vi "TC Channel Config.vi"(8 "error in (no error)":errorcluster, 11 "Node Ptr":T4 format="%.0x") -> (0 "error out":errorcluster)   [LabVIEW 2011, in "Simulated Thermocouple Custom Device.lvlib"]
uses:
  Simulated Thermocouple Custom Device.lvlib
  <vilib>/NI Veristand/Custom Device API/Custom Device Item Ref.ctl
  TC Channel Config Data.ctl
  TC Selector.ctl
  TC Unit Selector.ctl
  Calibration Config Data.ctl
  <vilib>/NI Veristand/Custom Device API/Get Item Property (Variant).vi
  <vilib>/NI Veristand/Custom Device API/Get Item Property (String).vi
  <vilib>/NI Veristand/Custom Device API/Set Item Property (String).vi
  <vilib>/NI Veristand/Custom Device API/Set Item Property (Variant).vi
  <vilib>/regexp/Match Regular Expression.xnode
  <vilib>/NI Veristand/Custom Device API/Custom Device API.lvlib
panel:
  out "Address":string
  in  "Physical Channel":u16(ring) items=["0", "1", "2", "3", "4", "5", "6", "7", "8", "9", "10", "11", "12", "13", "14", "15", "16", "17", "18", "19", "20", "21", "22", "23", "24", "25", "26", "27", "28", "29", "30", "31"]
  in  "Header 3":cluster{"Section Name":string}={"Section Name"="Physical Channel"}
  out "TC Channel Config":T1 {"Temperature Units" items=["Celcius", "Fahrenheit", "Kelvin", "Rankine", "Volts"]; "Thermocouple Type" items=["J", "K", "T", "E", "N", "B", "R", "S", "Raw Voltage"]}
  in  "Header 2":cluster{"Section Name":string}={"Section Name"="Thermocouple Settings"}
  in  "Header":cluster{"Section Name":string}={"Section Name"="Simulated Thermocouple Channel Specification"}
  in  "Description":string="This page allows you configure the type of thermocouple to simulate, and the units of the desired temperature output.  The phsyical channel below can be changed via the Physical Channel Selector."
  in  "Name":string
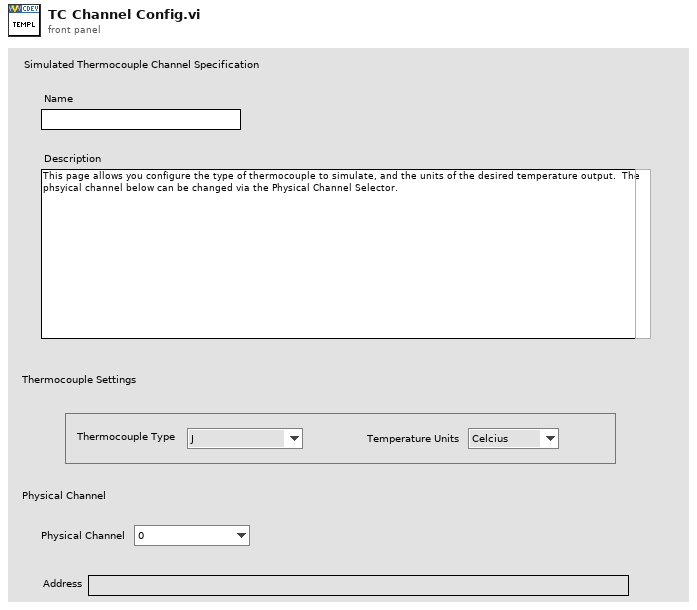
[diagram p1: front panel]
types:
  T1 = typedef "Simulated Thermocouple Custom Device.lvlib/TC Channel Config Data.ctl" = cluster{"Thermocouple Type":T2, "Temperature Units":T3}
  T2 = typedef "Simulated Thermocouple Custom Device.lvlib/TC Selector.ctl" = u16
  T3 = typedef "Simulated Thermocouple Custom Device.lvlib/TC Unit Selector.ctl" = u16
  T4 = typedef "Custom Device API.lvlib/Custom Device Item Ref.ctl" = u64
  T5 = typedef "Custom Device API.lvlib/Custom Device Item Info.ctl" = cluster{"Name":string, "Is Channel":bool, "GUID":string}
  T6 = typedef "Simulated Thermocouple Custom Device.lvlib/Calibration Config Data.ctl" = cluster{"Local SimTC Chan":string, "Samples To Collect":dbl, "Cal Channel TC Type":T2, "Cal Step Settling Time":dbl}
  T7 = typedef "Custom Device API.lvlib/Custom Device Commands.ctl" = enum16{"Default", "Item renamed", "Shutdown", "Dynamic button pressed"}
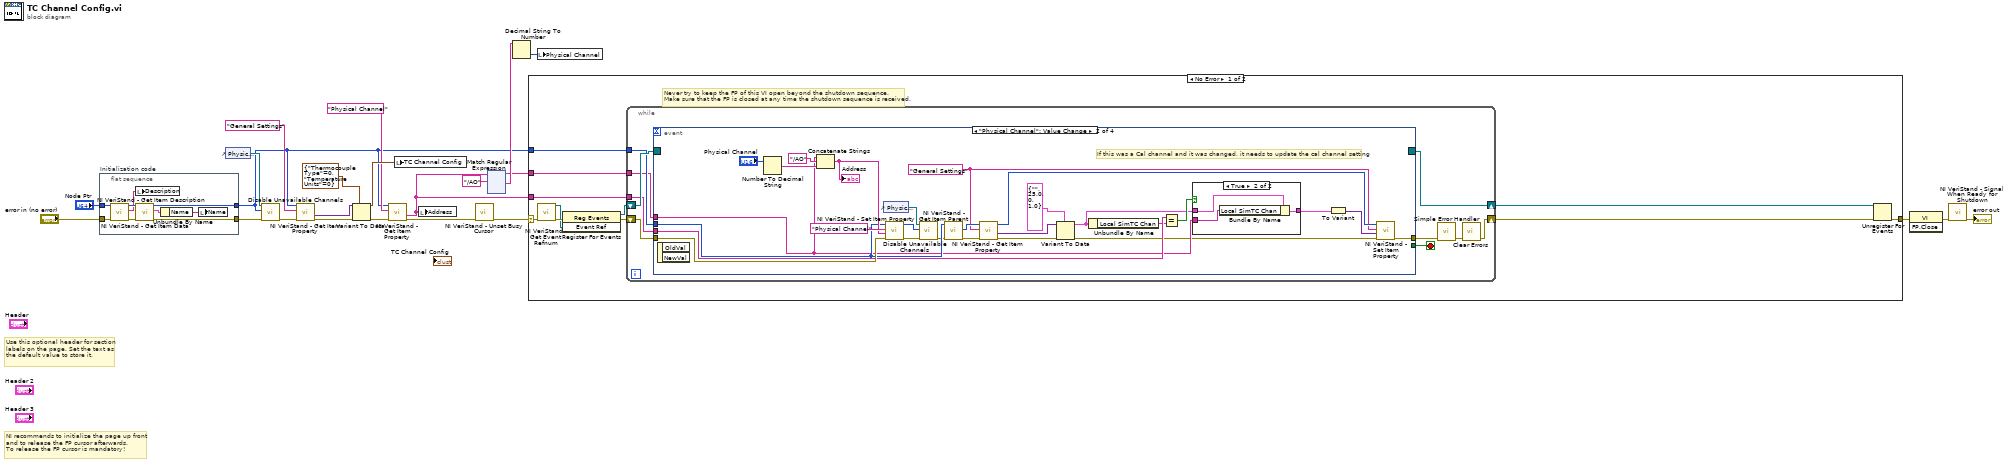
[diagram p0: block diagram]
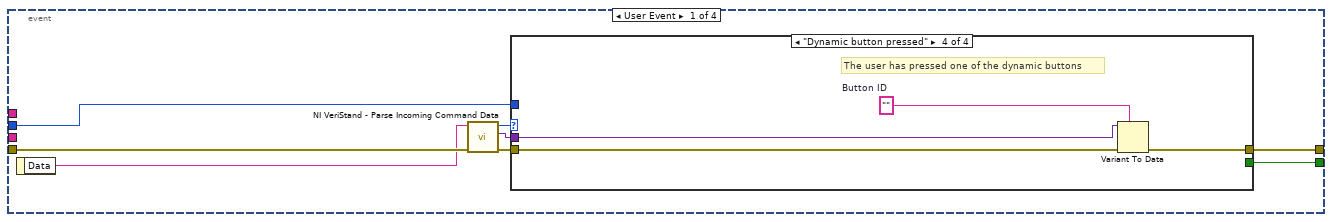
[diagram p2: hidden frame]
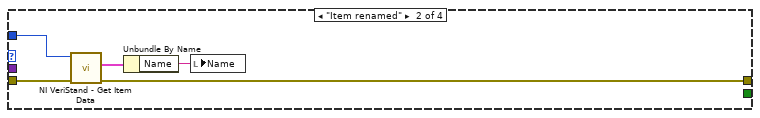
[diagram p4: hidden frame]
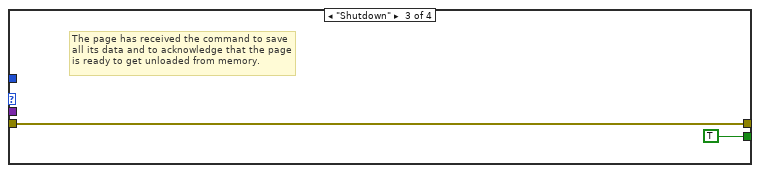
[diagram p5: hidden frame]
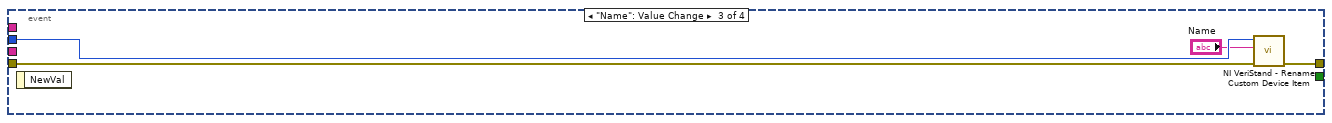
[diagram p7: hidden frame]
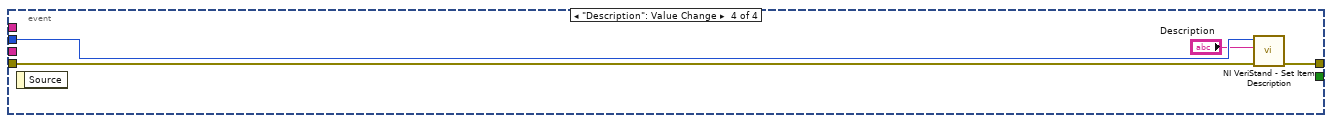
[diagram p8: hidden frame]
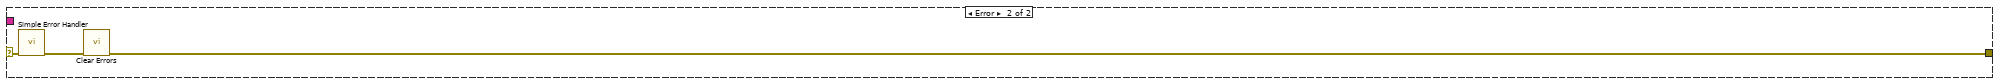
[diagram p9: hidden frame]
diagram:
  # "Use this optional header for section labels on the page. Set the text as the default value to store it."
  # "NI recommends to initialize the page up front\nand to release the FP cursor afterwards.\nTo release the FP cursor is mandatory!"
  n1 = flat-sequence "Initialization code" {
    tunnel: "error in (no error)" -> [w30]
    tunnel: "Node Ptr" -> [w29]
    tunnel: [w24] -> w17
    tunnel: [w32] -> w3
    frame #0 {
      n2 = call <vilib>:"NI VeriStand - Get Item Description.vi"("error in (no error)"=w30, "Item Ref in"=w29) -> ("error out"=w27:errorcluster, "Description"=w28:string, "Item Ref out"=w31:T4)  [unwired: 7 out]
      n3 = local write "Description"(w28) -> ()
      n4 = call <vilib>:"NI VeriStand - Get Item Data.vi"("error in (no error)"=w27, "Item Ref in"=w31) -> ("error out"=w24:errorcluster, "Item Info"=w26:T5, "Item Ref out"=w32:T4)  [unwired: 7 out]
      n5 = Unbundle By Name(w26) -> ("Name"=w25:string)
      n6 = local write "Name"(w25) -> ()
    }
  }
  n7 = control-ref of="Physical Channel"() -> (w16:refnum<vi>)
  n8 = call "Disable Unavailable Channels.vi"("error in (no error)"=w17, "Item Ref out"=w3, "Ring in"=w16) -> ("error out"=w15:errorcluster)  [unwired: 8 in]
  n9 = call-poly <vilib>:"NI VeriStand - Get Item Property.vi"("error in (no error)"=w15, "Property Name"="General Settings", "Item Ref in"=w3) -> ("error out"=w4:errorcluster, "Value"=w5:variant)  [unwired: 5 in, 2 out]
  n10 = Variant To Data(error in=w4, type=T1 {"Thermocouple Type"=0, "Temperature Units"=0} ("TC Channel Config"), Variant=w5) -> (data=w13:T1, error out=w12:errorcluster)
  n11 = call-poly <vilib>:"NI VeriStand - Get Item Property.vi"("error in (no error)"=w12, "Property Name"="Physical Channel", "Item Ref in"=w3) -> ("error out"=w8:errorcluster, "Value"=w1:string)  [unwired: 5 in, 2 out]
  n12 = local write "TC Channel Config"(w13) -> ()
  n13 = local write "Address"(w1) -> ()
  n14 = call <vilib>:"NI VeriStand - Unset Busy Cursor.vi"("error in (no error)"=w8) -> ("error out"=w19:errorcluster)  [unwired: 10 out]
  n15 = xnode "Match Regular Expression"("input string"=w1, "regular expression"="/AO") -> ("before match"=w7:string, "after match"=w10:string)  [unwired: 4 in, 3 out]
  n16 = Decimal String To Number(string=w10) -> (number=w9:i32)  [unwired: 2 in, 1 out]
  n17 = case shown="No Error" w19 {
    selector: w19 -> [w35 w115]
    tunnel: [w40 w113] -> w23
    tunnel: w3 -> [w36 _]
    tunnel: w7 -> [w34 _]
    tunnel: w1 -> [w33 _]
    frame No Error {
      # "Never try to keep the FP of this VI open beyond the shutdown sequence.\nMake sure that the FP is closed at any time the shutdown sequence is received."
      n18 = call <vilib>:"NI VeriStand - Get Event Refnum.vi"("error in (no error)"=w35) -> ("error out"=w43:errorcluster, "Event Ref"=w39:refnum<user-event>)  [unwired: 9 out]
      n19 = register-events(error in=w43, w39) -> (reference out=w37:refnum<event-registration>, error out=w38:errorcluster)  [unwired: 1 in]
      n20 = while {
        tunnel: w36 -> [w49]
        shift-right: [w46] -> w41
        shift-left: w38 -> [w52]
        shift-right: [w53] -> w42
        shift-left: w37 -> [w51]
        tunnel: w34 -> [w45]
        tunnel: w33 -> [w44]
        stop <- w50 stop-if-true
        n21 = event shown="[1] \"Physical Channel\": Value Change" {
          selector: w51 -> [_ _ _ _]
          dyn-events: [_ _ _ _] -> w53
          timeout: _ -> [_ _ _ _]
          tunnel: w52 -> [w61 w96 w108 w111]
          tunnel: [w57 _ _ _] -> w50
          tunnel: [w56 w76 w107 w110] -> w48
          tunnel: w49 -> [w55 w91 w106 w112]
          tunnel: w45 -> [_ w80 _ _]
          tunnel: w44 -> [_ w84 _ _]
          event User Event {
            n22 = event-data() -> ("Data"=w60:string)  [unwired: 1 out]
            n23 = call <vilib>:"NI VeriStand - Parse Incoming Command Data.vi"("error in (no error)"=w61, "Incoming data"=w60) -> ("error out"=w59:errorcluster, "Outgoing data"=w54:variant, "Action"=w58:T7)  [unwired: 7 out]
            n24 = case shown="\"Dynamic button pressed\"" w58 {
              tunnel: w59 -> [w62 w67 w68 w73]
              tunnel: [_ _ TRUE _] -> w57
              tunnel: [w62 w64 w68 w70] -> w56
              tunnel: w55 -> [_ w66 _ _]
              tunnel: w54 -> [_ _ _ w72]
              frame "Default", Default {
              }
              frame "Item renamed" {
                n25 = call <vilib>:"NI VeriStand - Get Item Data.vi"("error in (no error)"=w67, "Item Ref in"=w66) -> ("error out"=w64:errorcluster, "Item Info"=w65:T5)  [unwired: 8 out]
                n26 = Unbundle By Name(w65) -> ("Name"=w63:string)
                n27 = local write "Name"(w63) -> ()
              }
              frame "Shutdown" {
                # "The page has received the command to save all its data and to acknowledge that the page is ready to get unloaded from memory."
              }
              frame "Dynamic button pressed" {
                w71 = ""  # Button ID
                # "The user has pressed one of the dynamic buttons"
                n28 = Variant To Data(error in=w73, type=w71, Variant=w72) -> (error out=w70:errorcluster)  [unwired: 1 out]
              }
            }
          }
          event "Physical Channel": Value Change {
            w75 = "General Settings" ("Property Name")
            # "If this was a Cal channel and it was changed, it needs to update the cal channel setting"
            n29 = event-data() -> ()  [unwired: 3 out]
            n30 = Number To Decimal String(number="Physical Channel") -> (decimal integer string=w98:string)  [unwired: 1 in]
            n31 = Concatenate Strings(w80, "/AO" ("regular expression"), w98) -> (w95:string)
            "Address" <- w95
            n32 = control-ref of="Physical Channel"() -> (w93:refnum<vi>)
            n33 = call-poly <vilib>:"NI VeriStand - Set Item Property.vi"("error in (no error)"=w96, "Value"=w95, "Property Name"="Physical Channel", "Item Ref in"=w91) -> ("error out"=w92:errorcluster, "Item Ref out"=w94:T4)  [unwired: 5 in, 1 out]
            n34 = call "Disable Unavailable Channels.vi"("error in (no error)"=w92, "Item Ref out"=w94, "Ring in"=w93) -> ("error out"=w90:errorcluster)  [unwired: 8 in]
            n35 = call <vilib>:"NI VeriStand - Get Item Parent.vi"("error in (no error)"=w90, "Item Ref in"=w91) -> ("error out"=w87:errorcluster, "Parent Ref"=w89:T4)  [unwired: 6 in, 2 out]
            n36 = call-poly <vilib>:"NI VeriStand - Get Item Property.vi"("error in (no error)"=w87, "Property Name"=w75, "Item Ref in"=w89) -> ("error out"=w88:errorcluster, "Value"=w86:variant, "Item Ref out"=w79:T4)  [unwired: 5 in, 1 out]
            n37 = Variant To Data(error in=w88, type=T6 {"Local SimTC Chan"="", "Samples To Collect"=25.0, "Cal Channel TC Type"=0, "Cal Step Settling Time"=1.0} ("Cal Info"), Variant=w86) -> (data=w81:T6, error out=w77:errorcluster)
            n38 = Unbundle By Name(w81) -> ("Local SimTC Chan"=w83:string)
            n39 = Equal?(x=w84, y=w83) -> (x = y?=w82:bool)
            n40 = case shown="True" w82 {
              tunnel: w81 -> [w101 w104]
              tunnel: w80 -> [_ w103]
              tunnel: [w101 w102] -> w74
              frame False {
              }
              frame True {
                n41 = Bundle By Name(cluster=w104, "Local SimTC Chan"=w103) -> (w102:T6)
              }
            }
            n42 = To Variant(anything=w74) -> (Variant=w78:variant)
            n43 = call-poly <vilib>:"NI VeriStand - Set Item Property.vi"("error in (no error)"=w77, "Value"=w78, "Property Name"=w75, "Item Ref in"=w79) -> ("error out"=w76:errorcluster)  [unwired: 5 in, 2 out]
          }
          event "Name": Value Change {
            n44 = event-data() -> ()  [unwired: 2 out]
            n45 = call <vilib>:"NI VeriStand - Rename Custom Device Item.vi"("error in (no error)"=w108, "New Name"="Name", "Item Ref in"=w106) -> ("error out"=w107:errorcluster)  [unwired: 8 out]
          }
          event "Description": Value Change {
            n46 = event-data() -> ()  [unwired: 2 out]
            n47 = call <vilib>:"NI VeriStand - Set Item Description.vi"("error in (no error)"=w111, "Description"="Description", "Item Ref in"=w112) -> ("error out"=w110:errorcluster)  [unwired: 8 out]
          }
        }
        n48 = call <vilib>:"Simple Error Handler.vi"("error in (no error)"=w48) -> ("error out"=w47:errorcluster)  [unwired: 1 in, 7 out]
        n49 = call <vilib>:"Clear Errors.vi"("error in (no error)"=w47) -> ("error out"=w46:errorcluster)  [unwired: 6 out]
      }
      n50 = Unregister For Events(event registration refnum=w42, error in=w41) -> (error out=w40:errorcluster)
    }
    frame Error {
      n51 = call <vilib>:"Simple Error Handler.vi"("error in (no error)"=w115) -> ("error out"=w114:errorcluster)  [unwired: 1 in, 7 out]
      n52 = call <vilib>:"Clear Errors.vi"("error in (no error)"=w114) -> ("error out"=w113:errorcluster)  [unwired: 6 out]
    }
  }
  n53 = local write "Physical Channel"(w9) -> ()
  n54 = invoke class="VI" method="FP.Close"(error in=w23) -> (error out=w22:errorcluster)  [unwired: 2 in, 2 out]
  n55 = call <vilib>:"NI VeriStand - Signal When Ready for Shutdown.vi"("error in (no error)"=w22) -> ("error out"=→"error out":errorcluster)  [unwired: 10 out]
